vi "dfd_Moving Average G Check File Existence.vi"(6 "confirm?":bool=TRUE, 7 "# channels":i32=1, 8 "error in (no error)":errorcluster, 9 "filter name":string, 10 "dest path":path, 11 "MA filter":T1={"mMRate_Structure"=enum."CIC", "mMRate_Mode"=0, "mMRate_Factor"=1, "mMRate_FIRParams"={"mMRate_FIR_H"=[], "mMRate_FIR_IsNyquist?"=FALSE, "mMRate_FIR_IsSymmetric?"=FALSE}, "mMRate_CICParams"={"mMRate_CIC_#Stage"=2, "mMRate_CIC_Lag"=1, "mMRate_CIC_Type"=enum."Lowpass"}, "mMRate_Order"=0, "mMRate_Version"="1.0", "mMRate_Comments"="", "mMRate_RationalFactor"={"mMRate_L"=-1, "mMRate_M"=-1}, "mMRate_Fs"=1.0, "mMRate_Quantized?"=FALSE, "mMRate_QFilterGain"=1.0, "mMRate_CoefWl"=16, "mMRate_Scaling"={"mMRate_ScaleByPowerOf2?"=FALSE, "mMRate_ScaleType"=enum."Time Domain 1-Norm"}, "mMRate_InputWl"=0, "mMRate_OutputWl"=0, "mMRate_OutputMode"=enum."Nearest", "mMRate_MultMode"=enum."Full", "mMRate_BitPruning"=FALSE, "mMRate_GainWl"=16, "mMRate_OutputFwl"=0, "mMRate_SumIwl"=0, "mMRate_InputIwl "=16, "mMRate_SumWl"=32, "mMRate_CoefIwl"=0} {"mMRate_SumWl" min=1 max=32 step=1; "mMRate_InputIwl" min=1 max=32 step=1; "mMRate_GainWl" min=1 max=32 step=1; "mMRate_OutputWl" min=1 max=32 step=1; "mMRate_InputWl" min=1 max=32 step=1; "mMRate_CoefWl" min=1 max=32 step=1; "mMRate_Mode" items=["Default"=-1, "No Rate Change"=0, "Interpolation"=1, "Decimation"=2, "Interpolated"=3, "Rational"=4]}) -> (0 "error out":errorcluster, 1 "filter name out":string)   [LabVIEW 2017, in "NI_DigFilterLicensed.lvlib"]
uses:
  <vilib>/addons/Digital Filter Design/NI_DigFilterLicensed.lvlib
  <vilib>/addons/Digital Filter Design/_Objects.llb/DFD Multirate Filter Obj.ctl
  <vilib>/addons/Digital Filter Design/_Objects.llb/DFD Multirate Mode.ctl
  <vilib>/addons/Digital Filter Design/_Objects.llb/DFD Coef Norm Type.ctl
  <vilib>/addons/Digital Filter Design/_Objects.llb/DFD Round-off Mode.ctl
  <vilib>/addons/Digital Filter Design/_Objects.llb/DFD FXP MRate Multiply Mode.ctl
  <vilib>/addons/Digital Filter Design/_Misc.llb/dfd_Error Handlers (Single).vi
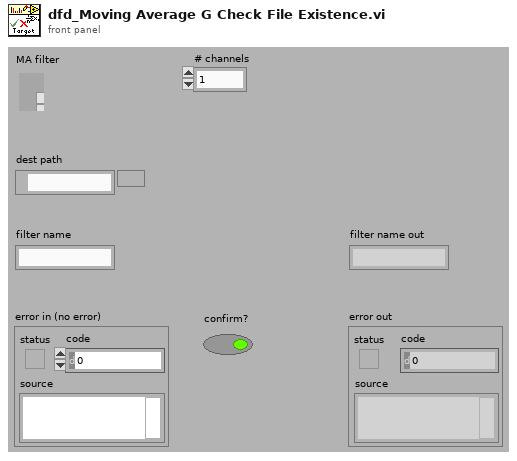
[diagram p1: front panel]
types:
  T1 = typedef "NI_DigFilterLicensed.lvlib/DFD Multirate Filter Obj.ctl" = cluster{"mMRate_Structure":enum16{"CIC", "FIR", "IIR", "Lattice"}, "mMRate_Mode":T2, "mMRate_Factor":i32, "mMRate_FIRParams":cluster{"mMRate_FIR_H":dbl[], "mMRate_FIR_IsNyquist?":bool, "mMRate_FIR_IsSymmetric?":bool}, "mMRate_CICParams":cluster{"mMRate_CIC_#Stage":i32, "mMRate_CIC_Lag":i32, "mMRate_CIC_Type":enum16{"Lowpass", "Highpass"}}, "mMRate_Order":i32, "mMRate_Version":string, "mMRate_Comments":string, "mMRate_RationalFactor":cluster{"mMRate_L":i32, "mMRate_M":i32}, "mMRate_Fs":dbl, "mMRate_Quantized?":bool, "mMRate_QFilterGain":dbl, "mMRate_CoefWl":i16, "mMRate_Scaling":cluster{"mMRate_ScaleByPowerOf2?":bool, "mMRate_ScaleType":T3}, "mMRate_InputWl":i16, "mMRate_OutputWl":i16, "mMRate_OutputMode":T4, "mMRate_MultMode":T5, "mMRate_BitPruning":bool, "mMRate_GainWl":i16, "mMRate_OutputFwl":i16, "mMRate_SumIwl":i16, "mMRate_InputIwl ":i16, "mMRate_SumWl":i16, "mMRate_CoefIwl":i16}
  T2 = typedef "NI_DigFilterLicensed.lvlib/DFD Multirate Mode.ctl" = i16
  T3 = typedef "NI_DigFilterLicensed.lvlib/DFD Coef Norm Type.ctl" = enum16{"No Norm", "Time Domain 1-Norm", "Time Domain 2-Norm", "Time Domain Inf-Norm"}
  T4 = typedef "NI_DigFilterLicensed.lvlib/DFD Round-off Mode.ctl" = enum16{"Nearest", "Truncation"}
  T5 = typedef "NI_DigFilterLicensed.lvlib/DFD FXP MRate Multiply Mode.ctl" = enum16{"Truncated", "Full"}
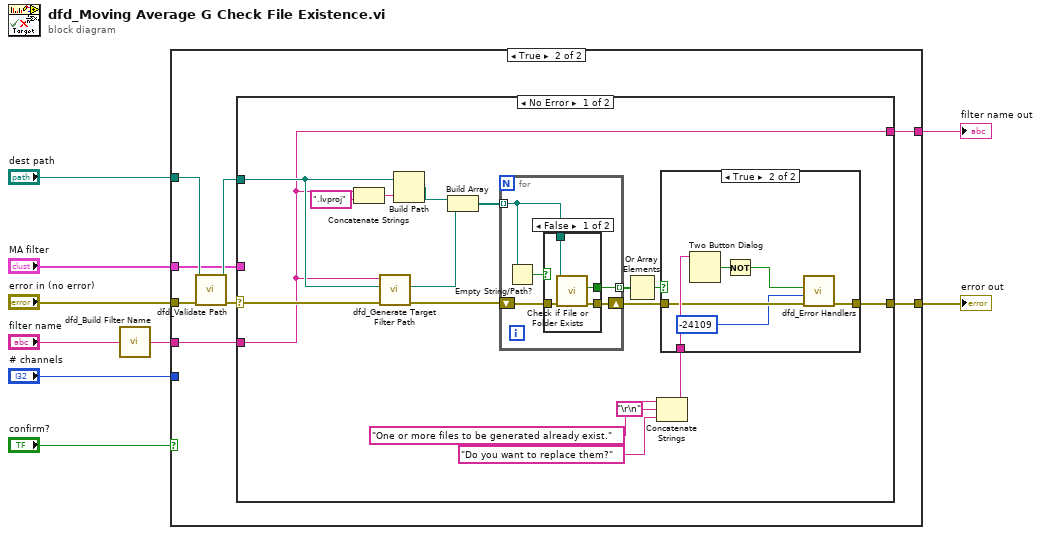
[diagram p0: block diagram]
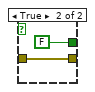
[diagram p4: hidden frame]
diagram:
  n1 = call <vilib>:"dfd_Build Filter Name.vi"("filter name in"="filter name") -> ("filter name out"=w1:string)
  n2 = case shown="True" "confirm?" {
    tunnel: "error in (no error)" -> [w10 w19]
    tunnel: "dest path" -> [_ w18]
    tunnel: w1 -> [w11 w17]
    tunnel: [w11 w15] -> w7
    tunnel: [w10 w13] -> w6
    tunnel: "MA filter" -> [_ w12]
    tunnel: "# channels" -> [_ _]
    frame False {
    }
    frame True {
      n3 = call <vilib>:"dfd_Validate Path.vi"("error in (no error)"=w19, "path in"=w18) -> ("error out"=w14:errorcluster, "path out"=w16:path)  [unwired: 8 out]
      n4 = case shown="No Error" w14 {
        selector: w14 -> [w24 w56]
        tunnel: w17 -> [w20 w55]
        tunnel: w16 -> [w22 _]
        tunnel: [w20 w55] -> w15
        tunnel: [w26 w56] -> w13
        tunnel: w12 -> [_ _]
        frame No Error {
          n5 = Concatenate Strings(w20, ".lvproj" ("string")) -> (w35:string)
          n6 = call <vilib>:"dfd_Generate Target Filter Path.vi"("error in (no error)"=w24, "destination path"=w22, "filter name"=w20) -> ("error out"=w23:errorcluster, "target VI path"=w21:path)  [unwired: 7 out]
          n7 = Build Path(base path=w22, name or relative path=w35) -> (appended path=w34:path)
          n8 = Build Array(w34, w21) -> (w25:path[])
          n9 = for {
            shift-right: [w47] -> w31
            shift-left: w23 -> [w48]
            tunnel: [w46] -> w33 mode=indexing
            tunnel: w25 -> [w44] mode=indexing
            n10 = Empty String/Path?(string/path=w44) -> (empty?=w45:bool)
            n11 = case shown="False" w45 {
              tunnel: w48 -> [w52 w53]
              tunnel: [w51 w53] -> w47
              tunnel: [w50 FALSE ("file or folder exists?")] -> w46
              tunnel: w44 -> [w49 _]
              frame False {
                n12 = call <vilib>:"Check if File or Folder Exists.vi"("error in (no error)"=w52, "path"=w49) -> ("error out"=w51:errorcluster, "file or folder exists?"=w50:bool)  [unwired: 8 out]
              }
              frame True {
              }
            }
          }
          n13 = Or Array Elements(Boolean array=w33) -> (logical OR=w32:bool)
          n14 = Concatenate Strings("One or more files to be generated already exist.", "\r\n", "Do you want to replace them?") -> (w27:string)
          n15 = case shown="True" w32 {
            tunnel: w31 -> [w37 w42]
            tunnel: w27 -> [_ w43]
            tunnel: [w37 w41] -> w26
            frame False {
            }
            frame True {
              n16 = Two Button Dialog(message=w43) -> (T button?=w40:bool)  [unwired: 2 out]
              n17 = Not(x=w40) -> (.not. x?=w39:bool)
              n18 = call-poly <vilib>:"dfd_Error Handlers.vi"("error in (no error)"=w42, "error code"=-24109 ("ERR_CODEGEN_CANCELLED"), "condition failed?"=w39) -> ("error out"=w41:errorcluster)  [unwired: 8 out]
            }
          }
        }
        frame Error {
        }
      }
    }
  }
  "error out" <- w6
  "filter name out" <- w7
